vi "Step 6.vi"(8 "error in (no error)":errorcluster, 11 "HeatUp Data in":string[][](array[string])) -> (0 "error out":errorcluster, 1 "T2-Setpoint":dbl[](graph), 2 "Raw Data":dbl[][](array[numeric]), 3 "Overshoot":dbl)   [LabVIEW 2016]
uses:
  <vilib>/Utility/error.llb/DialogType.ctl
panel:
  out "T2 Max":dbl
  out "T2":dbl[](graph)
  out "Setpoint":dbl[](graph)
  out "Setpoint Max":dbl
  out "Determine Time of UE Cutout":dbl
  out "HeatUp Data in 2":string[][](array[string])
  # "Data with Stripped Header"
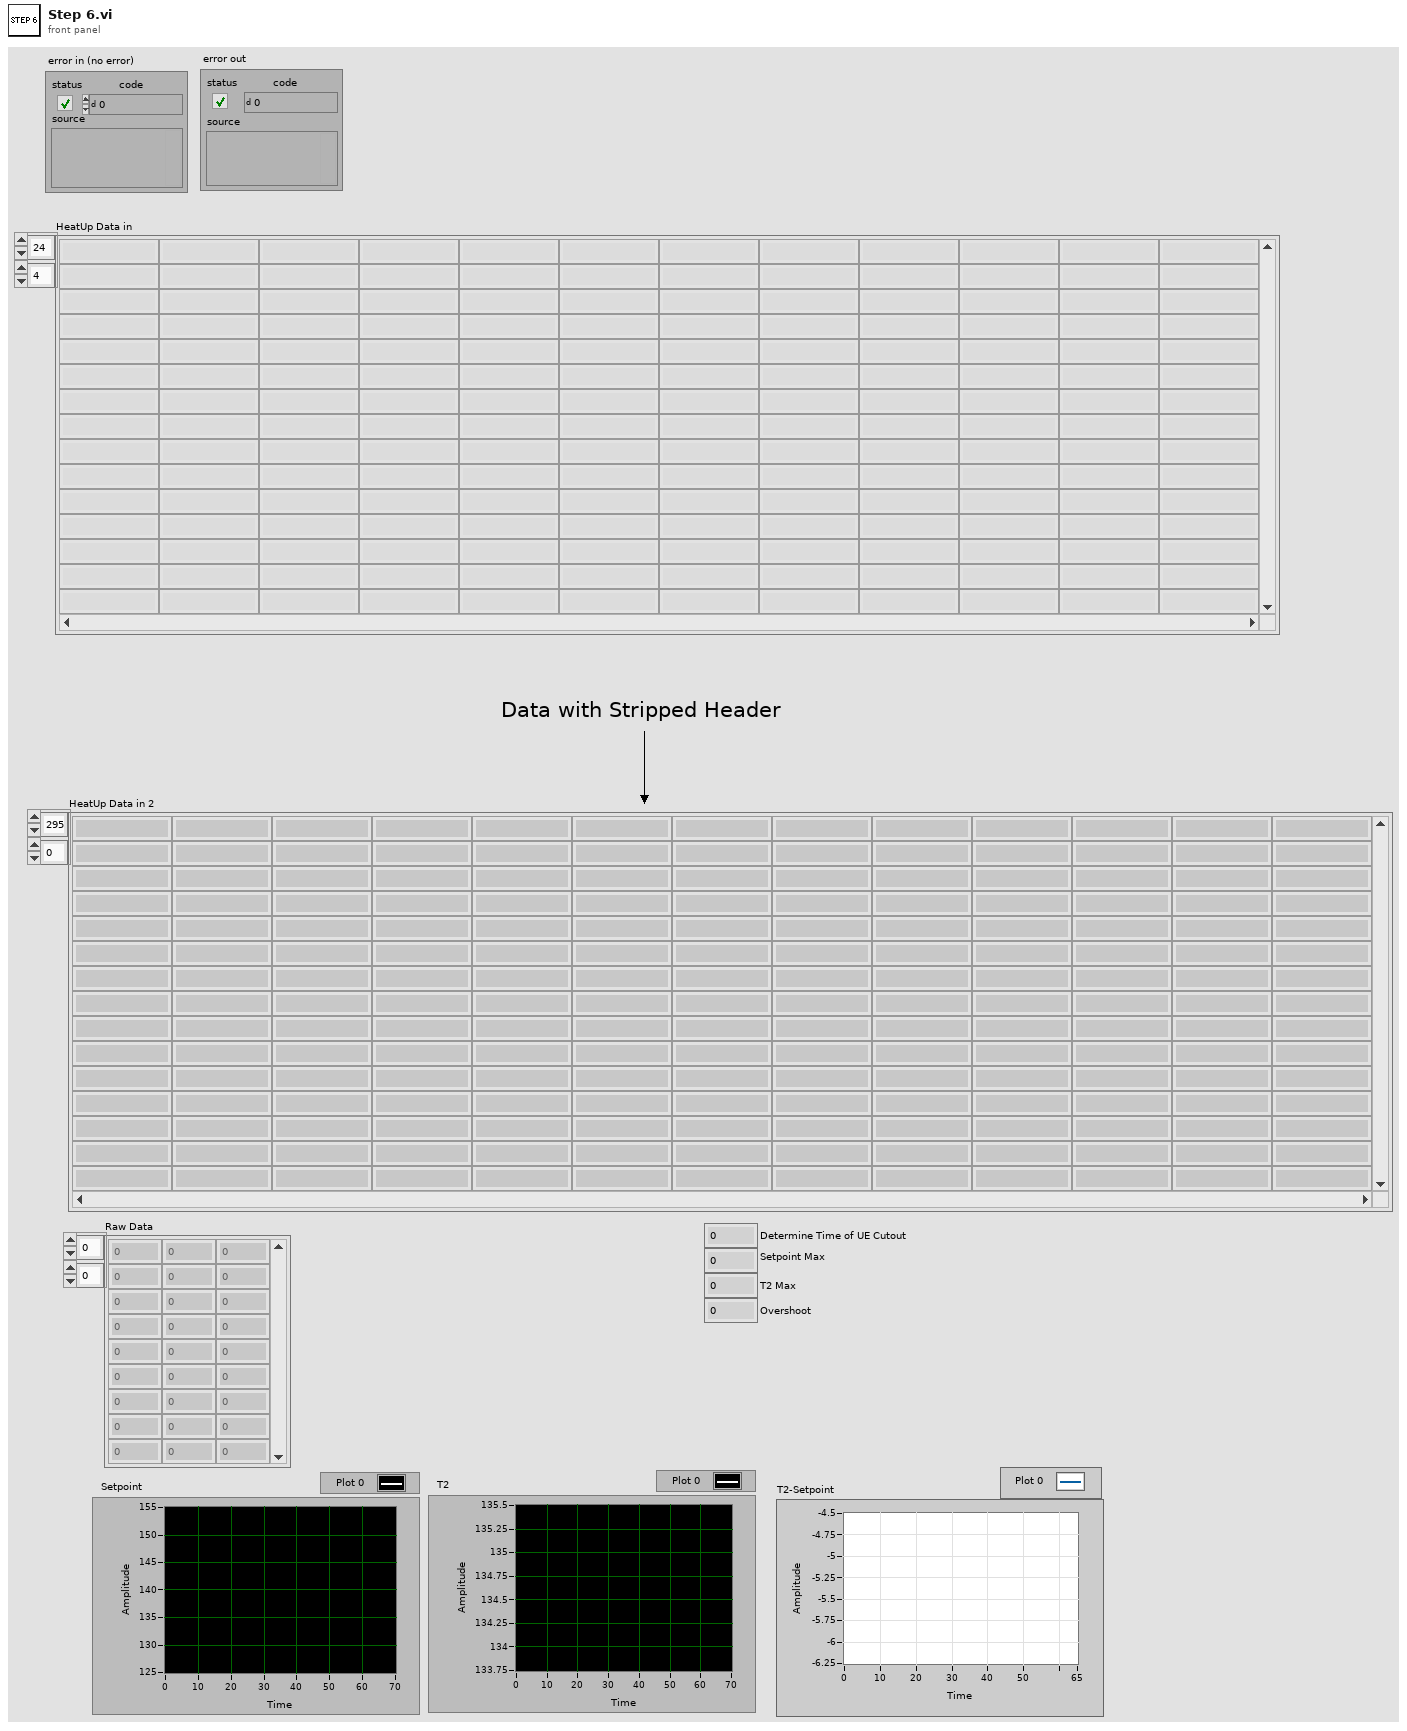
[diagram p1: front panel]
types:
  T1 = typedef "DialogType.ctl" = u16
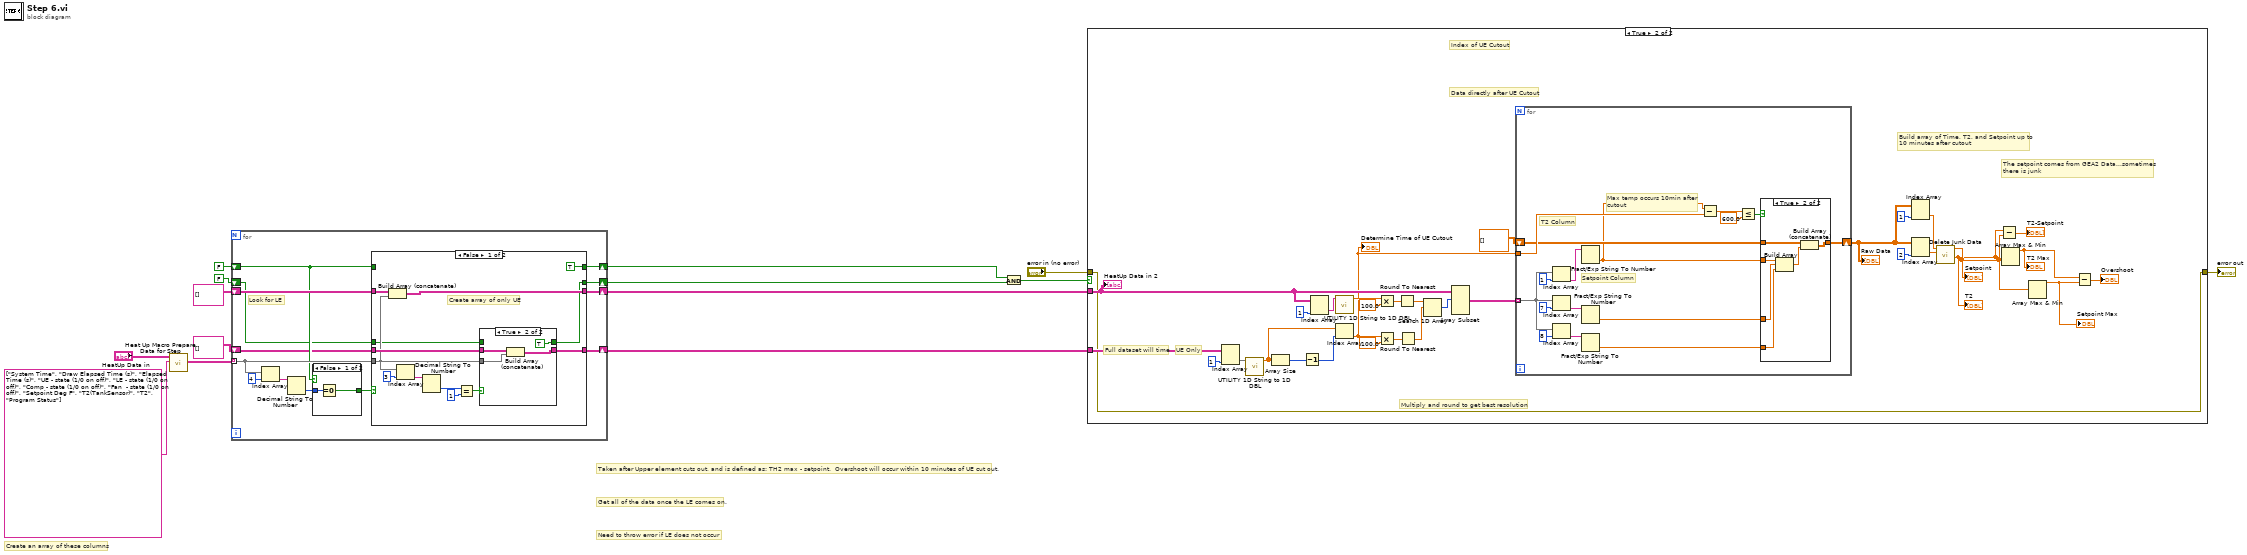
[diagram p0: block diagram]
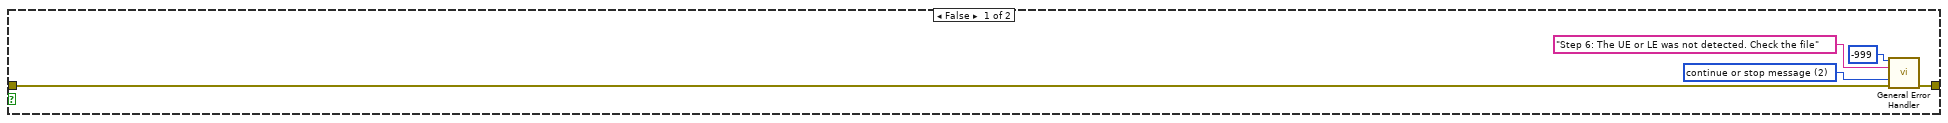
[diagram p2: hidden frame]
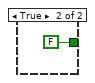
[diagram p4: hidden frame]
diagram:
  # "Need to throw error if LE does not occur"
  # "Get all of the data once the LE comes on."
  # "Taken after Upper element cuts out, and is defined as: TH2 max - setpoint.  Overshoot will occur within 10 minutes of UE cut out."
  # "Create an array of these columns"
  n1 = call "Heat Up Macro Prepare Data for Step.vi"("Columns Too Search For"=string[] ["System Time", "Draw Elapsed Time (s)", "Elapsed Time (s)", "UE - state (1/0 on off)", "LE - state (1/0 on off)", "Comp - state (1/0 on off)", "Fan  - state (1/0 on off)", "Setpoint Deg F", "T2(TankSensor)", "T2", "Program Status"], "HeatUp Raw Data Input"="HeatUp Data in") -> ("Heat Up Data with Only Selected Columns"=w1:string[][])  [unwired: 8 in, 1 out]
  n2 = for {
    tunnel: w1 -> [w25] mode=indexing
    shift-right: [w26] -> w9
    shift-left: string[][] [] -> [w27]
    shift-right: [w19] -> w7
    shift-left: FALSE -> [w20]
    shift-right: [w17] -> w10
    shift-left: string[][] [] -> [w18]
    shift-right: [w15] -> w6
    shift-left: FALSE -> [w16]
    # "Look for LE"
    n3 = Index Array(array=w25, index=4) -> (element=w23:string)
    n4 = Decimal String To Number(string=w23) -> (number=w22:i32)  [unwired: 2 in, 1 out]
    n5 = case shown="False" w20 {
      tunnel: w22 -> [w29 _]
      tunnel: [w28 FALSE] -> w21
      frame False {
        n6 = Equal To 0?(x=w29) -> (x = 0?=w28:bool)
      }
      frame True {
      }
    }
    n7 = case shown="False" w21 {
      tunnel: w27 -> [w43 w53]
      tunnel: [w41 w53] -> w26
      tunnel: w25 -> [w35 _]
      tunnel: w20 -> [_ w52]
      tunnel: [TRUE w52] -> w19
      tunnel: w18 -> [w40 w51]
      tunnel: [w39 w51] -> w17
      tunnel: w16 -> [w32 w50]
      tunnel: [w38 w50] -> w15
      frame False {
        # "Create array of only UE"
        n8 = Build Array (concatenate)(w43, w35) -> (w41:string[][])
        n9 = Index Array(array=w35, index=3) -> (element=w37:string)
        n10 = Decimal String To Number(string=w37) -> (number=w31:i32)  [unwired: 2 in, 1 out]
        n11 = Equal?(x=w31, y=1) -> (x = y?=w33:bool)
        n12 = case shown="True" w33 {
          tunnel: w40 -> [w45 w49]
          tunnel: [w45 w48] -> w39
          tunnel: w35 -> [_ w46]
          tunnel: [w44 TRUE] -> w38
          tunnel: w32 -> [w44 _]
          frame False {
          }
          frame True {
            n13 = Build Array (concatenate)(w49, w46) -> (w48:string[][])
          }
        }
      }
      frame True {
      }
    }
  }
  n14 = And(x=w7, y=w6) -> (x .and. y?=w8:bool)
  n15 = case shown="True" w8 {
    tunnel: w10 -> [_ w90]
    tunnel: w9 -> [_ w76]
    tunnel: "error in (no error)" -> [w58 w62]
    tunnel: [w57 w62] -> w4
    frame False {
      w56 = T1 2 items=["no dialog", "OK message", "continue or stop message", "OK message + warnings", "continue/stop + warnings"] ("type of dialog (OK msg:1)")
      n16 = call <vilib>:"General Error Handler.vi"("[error code] (0)"=-999, "[error source] (\" \")"="Step 6: The UE or LE was not detected. Check the file" ("[error source] (\" \")"), "type of dialog (OK msg:1)"=w56, "error in (no error)"=w58) -> ("error out"=w57:errorcluster)  [unwired: 7 in, 4 out]
    }
    frame True {
      # "Multiply and round to get best resolution"
      # "Full dataset will time"
      # "The setpoint comes from GEA2 Data...sometimes\nthere is junk"
      # "Index of UE Cutout"
      # "UE Only"
      # "Build array of Time, T2, and Setpoint up to\n10 minutes after cutout"
      # "Data directly after UE Cutout"
      n17 = Index Array(array=w90, index (col)=1 ("disabled index (col)")) -> (element=w88:string[])  [unwired: 1 in]
      n18 = call "UTILITY 1D String to 1D DBL.vi"("Save Data"=w88) -> ("DBL"=w87:dbl[])  [unwired: 10 in]
      n19 = Array Size(array=w87) -> (size(s)=w86:i32)
      n20 = Decrement(x=w86) -> (x-1=w85:i32)
      n21 = Index Array(array=w76, index (col)=1 ("disabled index (col)")) -> (element=w83:string[])  [unwired: 1 in]
      n22 = call "UTILITY 1D String to 1D DBL.vi"("Save Data"=w83) -> ("DBL"=w80:dbl[])  [unwired: 10 in]
      n23 = Index Array(array=w87, index=w85) -> (element=w63:dbl)
      "Determine Time of UE Cutout" <- w63
      n24 = Multiply(x=w80, y=100.0) -> (x*y=w78:dbl[])
      n25 = Multiply(x=w63, y=100.0) -> (x*y=w81:dbl)
      n26 = Round To Nearest(number=w78) -> (nearest integer value=w77:dbl[])
      n27 = Round To Nearest(number=w81) -> (nearest integer value=w73:dbl)
      n28 = Search 1D Array(1D array=w77, element=w73) -> (index of element=w75:i32)  [unwired: 1 in]
      n29 = Array Subset(array=w76, index (row)=w75) -> (w74:string[][])  [unwired: 3 in]
      n30 = for {
        tunnel: w74 -> [w95] mode=indexing
        tunnel: w63 -> [w104]
        shift-right: [w99] -> w69
        shift-left: dbl[][] [] -> [w100]
        # "Setpoint Column"
        # "T2 Column"
        # "Max temp occurs 10min after\ncutout"
        n31 = Index Array(array=w95, index=1 ("disabled index (col)")) -> (element=w105:string)
        n32 = Index Array(array=w95, index=7 ("disabled index (col)")) -> (element=w94:string)
        n33 = Index Array(array=w95, index=8 ("disabled index (col)")) -> (element=w93:string)
        n34 = Fract/Exp String To Number(string=w105) -> (number=w98:dbl)  [unwired: 3 in, 1 out]
        n35 = Fract/Exp String To Number(string=w94) -> (number=w92:dbl)  [unwired: 3 in, 1 out]
        n36 = Fract/Exp String To Number(string=w93) -> (number=w91:dbl)  [unwired: 3 in, 1 out]
        n37 = Subtract(x=w98, y=w104) -> (x-y=w103:dbl)
        n38 = Less Or Equal?(x=w103, y=600.0) -> (x <= y?=w101:bool)
        n39 = case shown="True" w101 {
          tunnel: w100 -> [w107 w113]
          tunnel: [w107 w112] -> w99
          tunnel: w98 -> [_ w111]
          tunnel: w92 -> [_ w110]
          tunnel: w91 -> [_ w109]
          frame False {
          }
          frame True {
            n40 = Build Array(w111, w110, w109) -> (w108:dbl[])
            n41 = Build Array (concatenate)(w113, w108) -> (w112:dbl[][])
          }
        }
      }
      "Raw Data" <- w69
      n42 = Index Array(array=w69, index (col)=1 ("disabled index (col)")) -> (element=w70:dbl[])  [unwired: 1 in]
      n43 = Index Array(array=w69, index (col)=2 ("disabled index (col)")) -> (element=w67:dbl[])  [unwired: 1 in]
      n44 = call "Delete Junk Data.vi"("DAQ Array"=w67, "Newfi Input Array"=w70) -> ("DAQ Array Output"=w60:dbl[], "Data"=w61:dbl[])  [unwired: 7 in, 1 out]
      "Setpoint" <- w61
      "T2" <- w60
      n45 = Subtract(x=w60, y=w61) -> (x-y=→"T2-Setpoint":dbl[])
      n46 = Array Max & Min(array=w60) -> (max value=w66:dbl)  [unwired: 3 out]
      "T2 Max" <- w66
      n47 = Array Max & Min(array=w61) -> (max value=w65:dbl)  [unwired: 3 out]
      "Setpoint Max" <- w65
      n48 = Subtract(x=w66, y=w65) -> (x-y=→"Overshoot":dbl)
      "HeatUp Data in 2" <- w76
    }
  }
  "error out" <- w4
